vi "PXI-Set Trigger Output.vi"(0 "Task in":refnum<k21>, 7 "Local Terminal Name":string="PXI_Trig4", 11 "error in (no error)":errorcluster) -> (4 "Task out":refnum<k21>, 6 "Trigger Terminal":string, 15 "error out":errorcluster)   [LabVIEW 2020]
uses:
  <resource>/objmgr/daqmx.rc
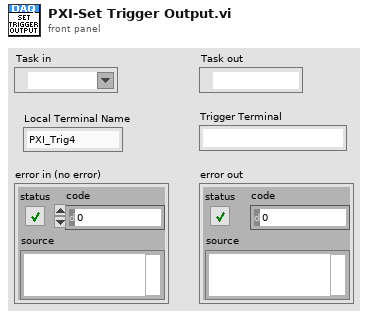
[diagram p1: front panel]
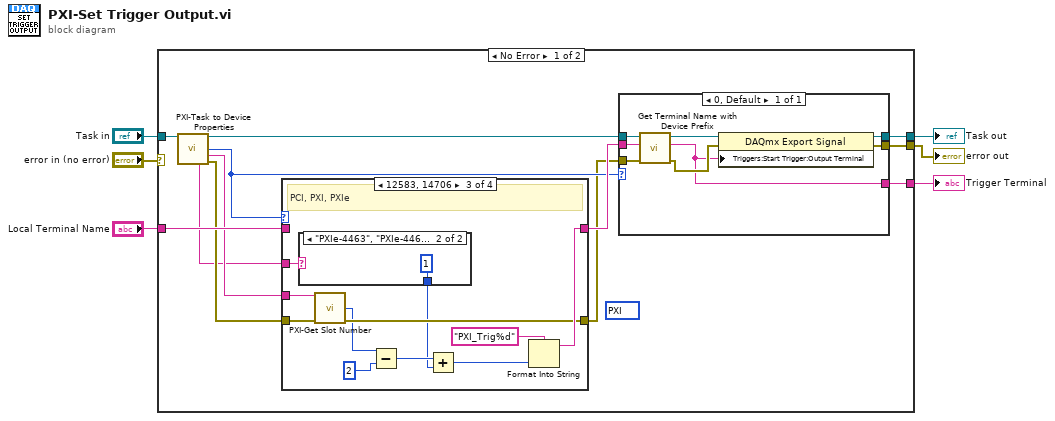
[diagram p0: block diagram]
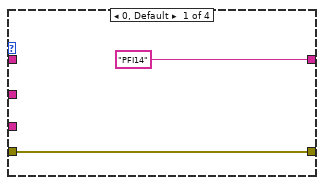
[diagram p2: hidden frame]
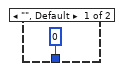
[diagram p4: hidden frame]
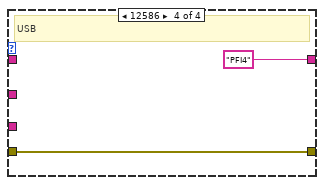
[diagram p5: hidden frame]
diagram:
  n1 = case shown="No Error" "error in (no error)" {
    selector: "error in (no error)" -> [_ w46]
    tunnel: "Task in" -> [w14 w47]
    tunnel: [w18 _] -> w4
    tunnel: [w17 w46] -> w5
    tunnel: [w16 w47] -> w6
    tunnel: "Local Terminal Name" -> [w11 _]
    frame No Error {
      (unwired) 12583 items=["PCI"=12582, "PCIe"=13612, "PXI"=12583, "PXIe"=14706, "SCXI"=12584, "SCC"=14707, "PCCard"=12585, "USB"=12586, "CompactDAQ"=14637, "TCP/IP"=14828, "Unknown"=12588, "SwitchBlock"=15870] ("BusType")
      n2 = call "PXI-Task to Device Properties.vi"("Task in"=w14) -> ("Task out"=w15:refnum<k21>, "BusType"=w12:i32, "Device"=w10:tag, "ProductType"=w7:string, "error out"=w9:errorcluster)  [unwired: 9 in, 1 out]
      n3 = case shown="12583, 14706" w12 {
        tunnel: ["PFI14" ("Local Terminal Name") w30 w37 "PFI4" ("Local Terminal Name")] -> w13
        tunnel: w11 -> [_ w30 _ _]
        tunnel: w10 -> [_ _ w36 _]
        tunnel: w9 -> [w27 w29 w35 w45]
        tunnel: [w27 w29 w34 w45] -> w8
        tunnel: w7 -> [_ _ w32 _]
        frame 0, Default {
        }
        frame 12582 {
          # "PCI"
        }
        frame 12583, 14706 {
          # "PCI, PXI, PXIe"
          n4 = case shown="\"PXIe-4463\", \"PXIe-4464\"" w32 {
            tunnel: [u32 0 ("y") u32 1 ("y")] -> w31
            frame "", Default {
            }
            frame "PXIe-4463", "PXIe-4464" {
            }
          }
          n5 = call "PXI-Get Slot Number.vi"("DAQmx Device Name in"=w36, "error in (no error)"=w35) -> ("Slot num"=w33:i32, "error out"=w34:errorcluster)  [unwired: 11 in, 1 out]
          n6 = Subtract(x=w33, y=2) -> (x-y=w40:i32)
          n7 = Add(x=w40, y=w31) -> (x+y=w39:u32)
          n8 = Format Into String(format string="PXI_Trig%d", w39) -> (resulting string=w37:string)  [unwired: 2 in, 1 out]
        }
        frame 12586 {
          # "USB"
        }
      }
      n9 = case shown="0, Default" w12 {
        tunnel: [w19] -> w18
        tunnel: [w24] -> w17
        tunnel: [w23] -> w16
        tunnel: w15 -> [w22]
        tunnel: w8 -> [w21]
        tunnel: w13 -> [w20]
        frame 0, Default {
          n10 = call "Get Terminal Name with Device Prefix.vi"("error in (no error)"=w21, "Local Terminal Name"=w20, "task/channels in"=w22) -> ("error out"=w26:errorcluster, "Terminal Name with Device Prefix"=w19:string, "task out"=w25:refnum<k21>)  [unwired: 6 in]
          n11 = property class="DAQmx Export Signal"(reference=w25, error in=w26, "Triggers:Start Trigger:Output Terminal"=w19) -> (reference out=w23:refnum<k21>, error out=w24:errorcluster)
        }
      }
    }
    frame Error {
    }
  }
  "Task out" <- w6
  "error out" <- w5
  "Trigger Terminal" <- w4
